vi "to_string.vi"(8 "error in (no error)":errorcluster, 11 "toml in":refnum<class "toml.lvclass">) -> (0 "error out":errorcluster, 2 "toml_string":string)   [LabVIEW 2020, in "toml.lvclass"]
uses:
  toml.lvclass
  toml.lvclass/toml.ctl
  Doc/Doc.lvclass
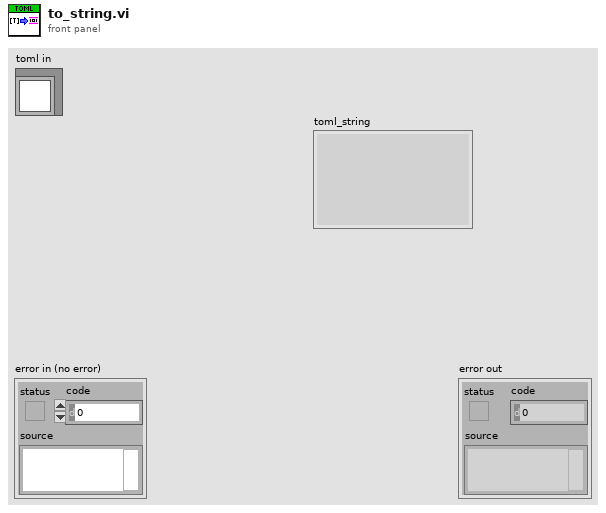
[diagram p1: front panel]
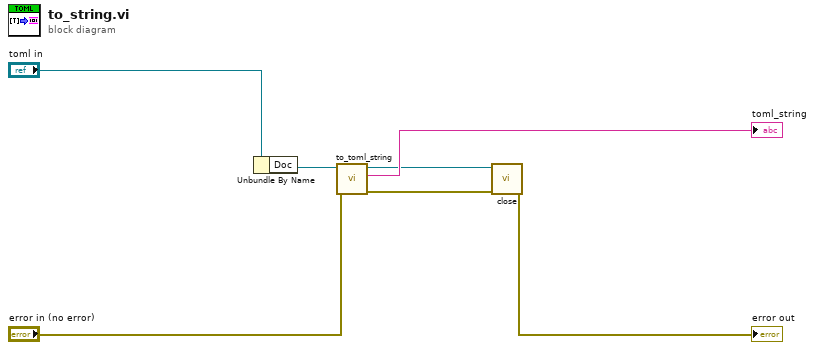
[diagram p0: block diagram]
diagram:
  n1 = Unbundle By Name("toml in") -> ("Doc"=w1:refnum<class "Doc.lvclass">)
  n2 = call "to_toml_string.vi"("error in (no error)"="error in (no error)", "Doc in"=w1) -> ("error out"=w2:errorcluster, "toml_string"=→"toml_string":string, "Doc out"=w3:refnum<class "Doc.lvclass">)  [unwired: 7 in]
  n3 = call "close.vi"("error in (no error)"=w2, "Doc in"=w3) -> ("error out"=→"error out":errorcluster)  [unwired: 9 in]
